vi "LDR Sensor ile LED Kontrolu.vi"() -> ()   [LabVIEW 2017]
uses:
  <vilib>/Instr/_visa.llb/VISA Configure Serial Port (Instr).vi
panel:
  out "Yüksek":bool
  in  "Yüksek":dbl
  in  "Normal":dbl
  out "Normal":bool
  out "Düþük":bool
  out "Gauge":dbl(knob) scale=0.0..700.0
  in  "stop":bool
  in  "Port COM":refnum<visa-resource-name>
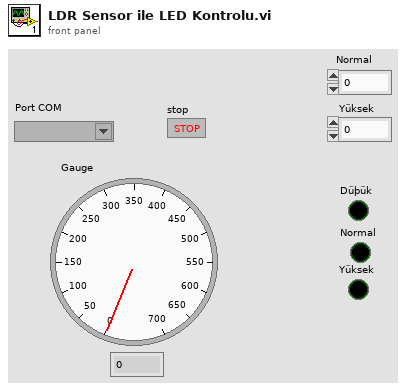
[diagram p1: front panel]
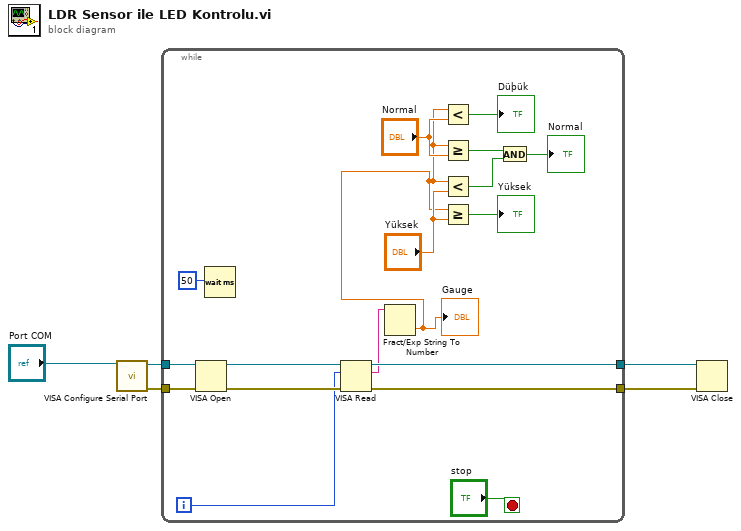
[diagram p0: block diagram]
diagram:
  n1 = call-poly "VISA Configure Serial Port"("VISA resource name"="Port COM") -> ("VISA resource name out"=w2:refnum<visa-resource-name>, "error out"=w5:errorcluster)  [unwired: 13 in]
  n2 = while {
    tunnel: w5 -> [w23]
    tunnel: [w21] -> w4
    tunnel: [w20] -> w3
    tunnel: w2 -> [w18]
    i -> [w15]
    stop <- "stop" stop-if-true
    n3 = VISA Open(error in (no error)=w23, VISA resource name=w18) -> (VISA resource name=w19:refnum<visa-resource-name>, error out=w22:errorcluster)  [unwired: 3 in]
    n4 = Wait (ms)(milliseconds to wait=u32 50 ("millisecond timer value")) -> ()  [unwired: 1 out]
    n5 = VISA Read(VISA resource name=w19, byte count=w15, error in (no error)=w22) -> (VISA resource name out=w20:refnum<visa-resource-name>, read buffer=w16:string, error out=w21:errorcluster)  [unwired: 1 out]
    n6 = Fract/Exp String To Number(string=w16) -> (number=w6:dbl)  [unwired: 3 in, 1 out]
    "Gauge" <- w6
    n7 = Less?(x=w6, y="Normal") -> (x < y?=→"Düþük":bool)
    n8 = Greater Or Equal?(x=w6, y="Normal") -> (x >= y?=w11:bool)
    n9 = Less?(x=w6, y="Yüksek") -> (x < y?=w10:bool)
    n10 = Greater Or Equal?(x=w6, y="Yüksek") -> (x >= y?=→"Yüksek":bool)
    n11 = And(x=w11, y=w10) -> (x .and. y?=→"Normal":bool)
  }
  n12 = VISA Close(VISA resource name=w3, error in (no error)=w4) -> ()  [unwired: 1 out]
